vi "absCalc.vi"(8 "Calibrant xssc (cm^2/molec)":dbl, 9 "[Calibrant] (molec/cc)":dbl, 10 "calibrant flows (sccm)":dbl[](array[numeric]), 11 "dilution flows (sccm)":dbl[](array[numeric])) -> (3 "Abs (1/Mm)":dbl[](array[numeric]))   [LabVIEW 2011]
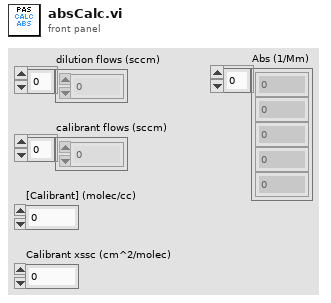
[diagram p1: front panel]
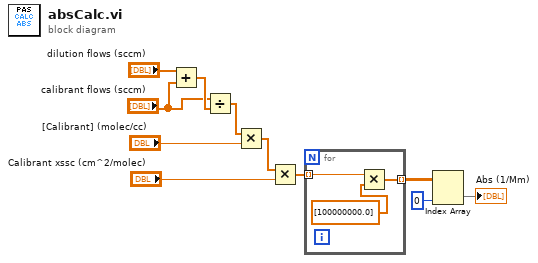
[diagram p0: block diagram]
diagram:
  n1 = Add(x="dilution flows (sccm)", y="calibrant flows (sccm)") -> (x+y=w6:dbl[])
  n2 = Divide(x="calibrant flows (sccm)", y=w6) -> (x/y=w7:dbl[])
  n3 = Multiply(x=w7, y="[Calibrant] (molec/cc)") -> (x*y=w9:dbl[])
  n4 = Multiply(x=w9, y="Calibrant xssc (cm^2/molec)") -> (x*y=w4:dbl[])
  n5 = for {
    tunnel: [w14] -> w3 mode=indexing
    tunnel: w4 -> [w13] mode=indexing
    n6 = Multiply(x=w13, y=dbl[] [100000000.0]) -> (x*y=w14:dbl[])
  }
  n7 = Index Array(array=w3, index (col)=0 ("disabled index (col)")) -> (element=→"Abs (1/Mm)":dbl[])  [unwired: 1 in]
